vi "Creat unit normal.vi"(1 "E2":sgl[](array[numeric]), 2 "E1":sgl[](array[numeric])) -> (0 "n^ = (E1 x E2) / ||E1 x E2||":sgl[](array[numeric]))   [LabVIEW 2014]
uses:
  Subroutines/Dot product.vi
panel:
  # "PN 17/03/2015"
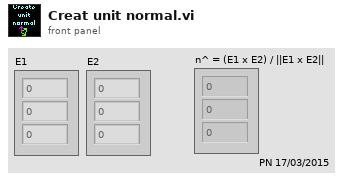
[diagram p1: front panel]
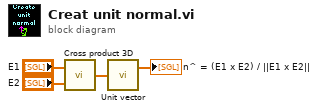
[diagram p0: block diagram]
diagram:
  n1 = call "Cross product 3D.vi"("B"="E2", "A"="E1") -> ("A x B"=w4:sgl[])
  n2 = call "Unit vector.vi"("Vector"=w4) -> ("Unit vector"=→"n^ = (E1 x E2) / ||E1 x E2||":sgl[])  [unwired: 1 out]
